vi "Prepare - Create Error if unable to load Subpanel.vi"(8 "error in (no error)":errorcluster) -> (0 "error out":errorcluster)   [LabVIEW 2022 SP3, in "UI Manager.lvlib"]
doc: "____\nHAMPEL SOFTWARE ENGINEERING v2.6.0 (2023-12-19 10:54)"
uses:
  UI Manager.lvlib
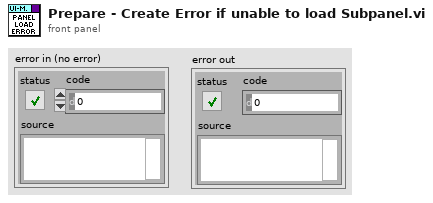
[diagram p1: front panel]
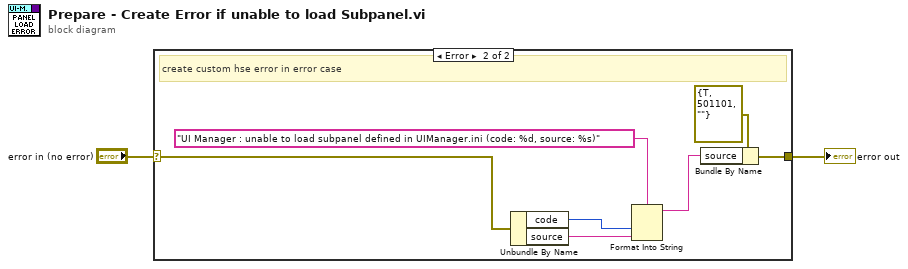
[diagram p0: block diagram]
diagram:
  n1 = case shown="Error" "error in (no error)" {
    selector: "error in (no error)" -> [w3 w7]
    tunnel: [w3 w6] -> w1
    frame No Error {
    }
    frame Error {
      # "create custom hse error in error case"
      n2 = Unbundle By Name(w7) -> ("code"=w9:i32, "source"=w4:string)
      n3 = Format Into String(format string="UI Manager : unable to load subpanel defined in UIManager.ini (code: %d, source: %s)", w9, w4) -> (resulting string=w5:string)  [unwired: 2 in, 1 out]
      n4 = Bundle By Name(cluster=errorcluster {"status"=TRUE, "code"=501101, "source"=""} ("error out"), "source"=w5) -> (w6:errorcluster)
    }
  }
  "error out" <- w1
